vi "Create Array if Repeating.vi"(6 "Location (0,0)":T1, 8 "error in (no error)":errorcluster, 9 "Label":string, 10 "Repeating":bool, 11 "Owner in":refnum<vi>) -> (0 "error out":errorcluster, 1 "Nested Label":string, 3 "Subcontrol Owner":refnum<vi>)   [LabVIEW 2024, in "LV-Protoc.lvlib"]
uses:
  LV-Protoc.lvlib
  <vilib>/Utility/miscctls.llb/LVPointTypeDef.ctl
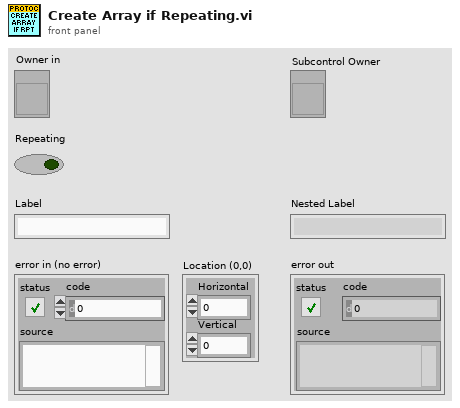
[diagram p1: front panel]
types:
  T1 = typedef "LVPointTypeDef.ctl" = cluster{"Horizontal":i16, "Vertical":i16}
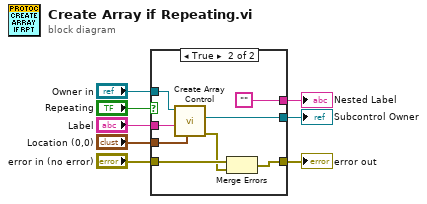
[diagram p0: block diagram]
diagram:
  n1 = case shown="True" "Repeating" {
    tunnel: "Owner in" -> [w10 w18]
    tunnel: "Location (0,0)" -> [_ w17]
    tunnel: "Label" -> [w9 w19]
    tunnel: "error in (no error)" -> [w11 w16]
    tunnel: [w11 w14] -> w3
    tunnel: [w10 w13] -> w2
    tunnel: [w9 "" ("Label")] -> w1
    frame False {
    }
    frame True {
      n2 = call "Create Array Control.vi"("Location (0,0)"=w17, "Label"=w19, "Owner in"=w18) -> ("error out"=w15:errorcluster, "Array Control"=w13:refnum<vi>)  [unwired: 7 in]
      n3 = Merge Errors(w16, w15) -> (w14:errorcluster)
    }
  }
  "error out" <- w3
  "Subcontrol Owner" <- w2
  "Nested Label" <- w1
